vi "Simple Example.vi"() -> ()   [LabVIEW 2011]
uses:
  Dictionary.lvlib
  Set/Set (DBL).vi
  Get/Get (DBL).vi
panel:
  out "Keys":string[](array[string])
  out "Values":string[](array[string])
  in  "stop":bool
  out "value":dbl
  out "found":bool
  in  "Key":string
  in  "Items":u16=1000
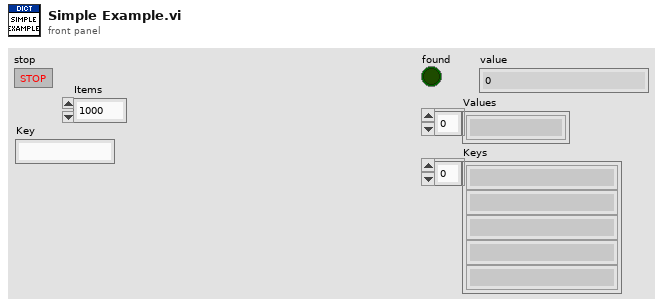
[diagram p1: front panel]
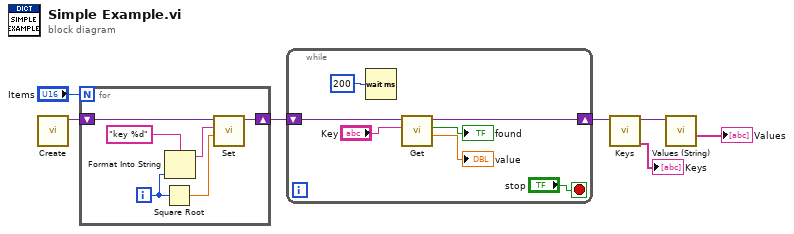
[diagram p0: block diagram]
diagram:
  n1 = call "Create.vi"() -> ("Dictionary"=w6:variant)  [unwired: 11 in]
  n2 = for {
    N: "Items" -> [_]
    shift-right: [w12] -> w5
    shift-left: w6 -> [w13]
    i -> [w9]
    n3 = Square Root(x=w9) -> (sqrt(x)=w8:dbl)
    n4 = Format Into String(format string="key %d", w9) -> (resulting string=w10:string)  [unwired: 2 in, 1 out]
    n5 = call-poly "Set.vi"("Value"=w8, "Key"=w10, "Dictionary in"=w13) -> ("Dictionary out"=w12:variant)  [unwired: 7 in, 1 out]
  }
  n6 = while {
    shift-right: [w18] -> w4
    shift-left: w5 -> [w20]
    stop <- "stop" stop-if-true
    n7 = Wait (ms)(milliseconds to wait=u32 200) -> ()  [unwired: 1 out]
    n8 = call-poly "Get.vi"("Key"="Key", "Dictionary in"=w20) -> ("value"=→"value":dbl, "found"=→"found":bool, "Dictionary out"=w18:variant)  [unwired: 7 in]
  }
  n9 = call "Keys.vi"("Dictionary in"=w4) -> ("Keys"=→"Keys":string[], "Dictionary out"=w3:variant)  [unwired: 9 in]
  n10 = call "Values (String).vi"("Dictionary in"=w3) -> ("Values"=→"Values":string[])  [unwired: 9 in, 1 out]
